vi "Create DB.vi"() -> ()   [LabVIEW 2015]
doc: "Drops any existing data from the test database and sets up tables for use in the project examples."
uses:
  <vilib>/drjdpowell/SQLite Library/SQL Connection/Open (string).vi
  <vilib>/drjdpowell/SQLite Library/SQL Connection/Connection.lvclass
panel:
  out "error out":errorcluster
  # "Drops any existing data from the test database and sets up tables for use in the project examples."
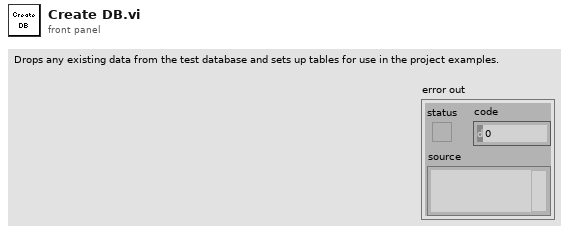
[diagram p1: front panel]
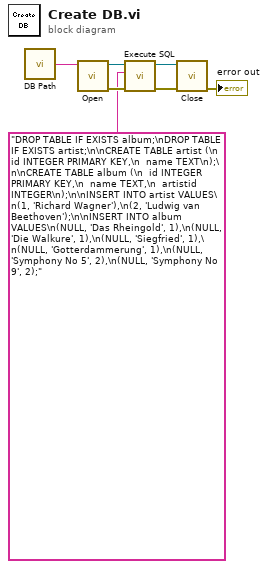
[diagram p0: block diagram]
diagram:
  n1 = call "DB Path.vi"() -> ("DB Path"=w4:string)
  n2 = call-poly <vilib>:"Open.vi"("db file"=w4) -> ("error out"=w6:errorcluster, "SQLite Connection"=w7:refnum<class "Connection.lvclass">)  [unwired: 9 in]
  n3 = call <vilib>:"Execute SQL.vi"("error in (no error)"=w6, "SQL"="DROP TABLE IF EXISTS album;\nDROP TABLE IF EXISTS artist;\n\nCREATE TABLE artist (\n  id INTEGER PRIMARY KEY,\n  name TEXT\n);\n\nCREATE TABLE album (\n  id INTEGER PRIMARY KEY,\n  name TEXT,\n  artistid INTEGER\n);\n\nINSERT INTO artist VALUES\n(1, 'Richard Wagner'),\n(2, 'Ludwig van Beethoven');\n\nINSERT INTO album VALUES\n(NULL, 'Das Rheingold', 1),\n(NULL, 'Die Walkure', 1),\n(NULL, 'Siegfried', 1),\n(NULL, 'Gotterdammerung', 1),\n(NULL, 'Symphony No 5', 2),\n(NULL, 'Symphony No 9', 2);", "SQLite Connection in"=w7) -> ("error out"=w1:errorcluster, "SQLite Connection"=w2:refnum<class "Connection.lvclass">)  [unwired: 5 in, 2 out]
  n4 = call-dynamic "Close.vi"("error in (no error)"=w1, "SQLite Connection in"=w2) -> ("error out"=→"error out":errorcluster)  [unwired: 9 in]
